vi "RSC_Generate_SubCondition_text.vi"(8 "error in (no error)":errorcluster, 10 "SubCondition #":i32, 11 "Subcondition":refnum<class "Reward_SubCondition.lvclass">) -> (0 "error out":errorcluster, 2 "Validity Criteria":string, 3 "Condition Info":string)   [LabVIEW 2018, in "Tracker.lvlib" / "Reward_SubCondition.lvclass"]
uses:
  Reward_SubCondition.lvclass
  Reward_SubCondition.lvclass/Reward_SubCondition.ctl
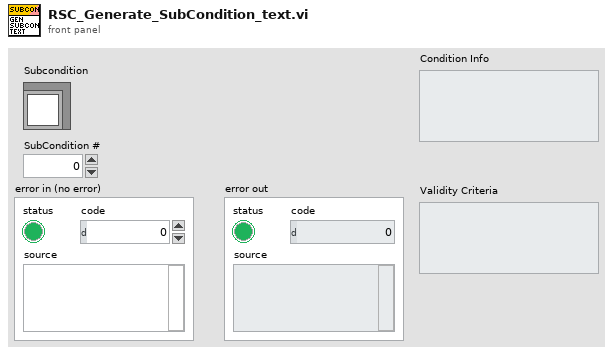
[diagram p1: front panel]
types:
  T1 = enum16{"Less", "Less or Equal", "Equal", "Greater or Equal", "Greater", "Not Equal"}
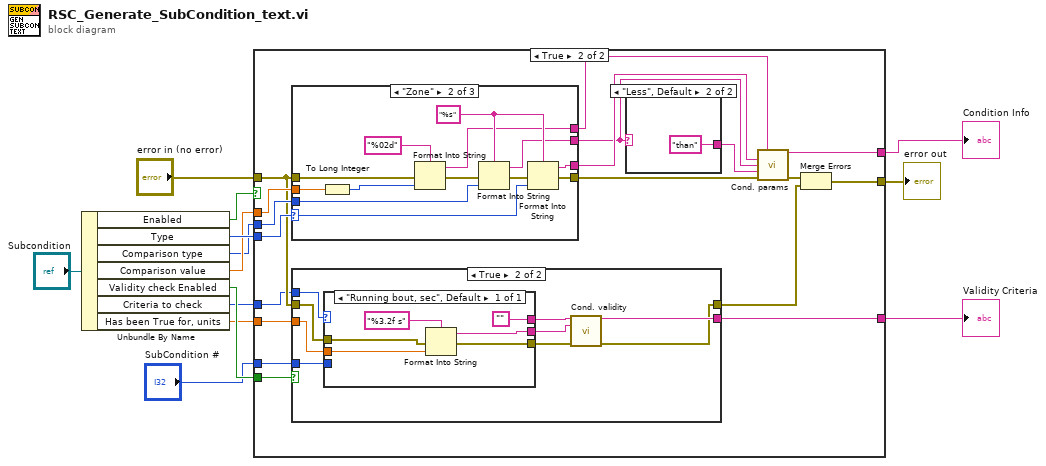
[diagram p0: block diagram]
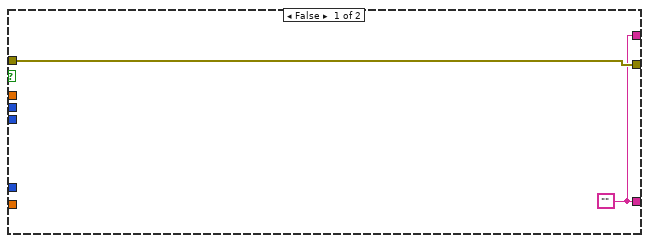
[diagram p2: hidden frame]
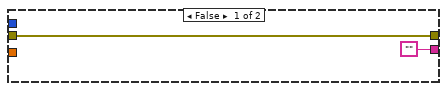
[diagram p3: hidden frame]
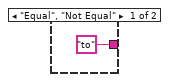
[diagram p4: hidden frame]
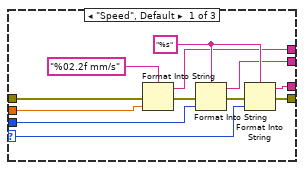
[diagram p5: hidden frame]
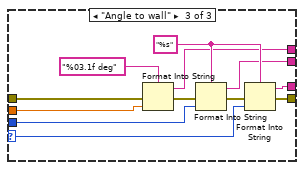
[diagram p6: hidden frame]
diagram:
  n1 = Unbundle By Name("Subcondition") -> ("Enabled"=w7:bool, "Type"=w11:enum16{"Angle to wall", "Speed", "Zone"}, "Comparison type"=w9:T1, "Comparison value"=w10:dbl, "Validity check Enabled"=w8:bool, "Criteria to check"=w4:enum16{"Running bout, sec", "Running bout, m"}, "Has been True for, units"=w5:dbl)
  n2 = case shown="True" w7 {
    tunnel: w11 -> [_ w33]
    tunnel: w10 -> [_ w32]
    tunnel: "error in (no error)" -> [w15 w28]
    tunnel: w9 -> [_ w31]
    tunnel: [w15 w22] -> w12
    tunnel: [w14 w17] -> w1
    tunnel: w8 -> [_ w19]
    tunnel: [w14 w27] -> w2
    tunnel: w5 -> [_ w21]
    tunnel: w4 -> [_ w20]
    tunnel: "SubCondition #" -> [_ w18]
    frame False {
      w14 = ""
    }
    frame True {
      n3 = case shown="\"Zone\"" w33 {
        selector: w33 -> [w62 w75 w88]
        tunnel: w32 -> [w63 w76 w82]
        tunnel: w28 -> [w60 w73 w86]
        tunnel: w31 -> [w61 w74 w87]
        tunnel: [w56 w65 w78] -> w25
        tunnel: [w55 w66 w79] -> w24
        tunnel: [w54 w67 w80] -> w26
        tunnel: [w53 w68 w81] -> w30
        frame "Speed", Default {
          w57 = "%s" ("format string")
          n4 = Format Into String(format string="%02.2f mm/s", error in=w60, w63) -> (resulting string=w54:string, error out=w59:errorcluster)  [unwired: 1 in]
          n5 = Format Into String(format string=w57, error in=w59, w61) -> (resulting string=w55:string, error out=w58:errorcluster)  [unwired: 1 in]
          n6 = Format Into String(format string=w57, error in=w58, w62) -> (resulting string=w56:string, error out=w53:errorcluster)  [unwired: 1 in]
        }
        frame "Zone" {
          w70 = "%s" ("format string")
          n7 = To Long Integer(number=w76) -> (32bit integer=w69:i32)
          n8 = Format Into String(format string="%02d", error in=w73, w69) -> (resulting string=w67:string, error out=w72:errorcluster)  [unwired: 1 in]
          n9 = Format Into String(format string=w70, error in=w72, w74) -> (resulting string=w66:string, error out=w71:errorcluster)  [unwired: 1 in]
          n10 = Format Into String(format string=w70, error in=w71, w75) -> (resulting string=w65:string, error out=w68:errorcluster)  [unwired: 1 in]
        }
        frame "Angle to wall" {
          w83 = "%s" ("format string")
          n11 = Format Into String(format string="%03.1f deg", error in=w86, w82) -> (resulting string=w80:string, error out=w85:errorcluster)  [unwired: 1 in]
          n12 = Format Into String(format string=w83, error in=w85, w87) -> (resulting string=w79:string, error out=w84:errorcluster)  [unwired: 1 in]
          n13 = Format Into String(format string=w83, error in=w84, w88) -> (resulting string=w78:string, error out=w81:errorcluster)  [unwired: 1 in]
        }
      }
      n14 = case shown="True" w19 {
        tunnel: w28 -> [w35 w44]
        tunnel: ["" w43] -> w17
        tunnel: [w35 w42] -> w16
        tunnel: w21 -> [_ w41]
        tunnel: w20 -> [_ w40]
        tunnel: w18 -> [_ w38]
        frame False {
        }
        frame True {
          n15 = case shown="\"Running bout, sec\", Default" w40 {
            tunnel: w44 -> [w48]
            tunnel: w41 -> [w49]
            tunnel: [w45] -> w39
            tunnel: [w47] -> w36
            tunnel: w38 -> [_]
            tunnel: [""] -> w37
            frame "Running bout, sec", Default {
              n16 = Format Into String(format string="%3.2f s", error in=w48, w49) -> (resulting string=w47:string, error out=w45:errorcluster)  [unwired: 1 in]
            }
          }
          n17 = call "Cond. validity"("Beginning Text"=w37, "value"=w36, "error in (no error)"=w39) -> ("Result"=w43:string, "error out"=w42:errorcluster)  [unwired: 11 in]
        }
      }
      n18 = case shown="\"Less\", Default" w24 {
        tunnel: ["to" "than"] -> w23
        frame "Equal", "Not Equal" {
        }
        frame "Less", Default {
        }
      }
      n19 = call "Cond. params"("comvalue"=w26, "condname"=w25, "comptype"=w24, "tie"=w23, "error in (no error)"=w30) -> ("Result"=w27:string, "error out"=w29:errorcluster)  [unwired: 9 in]
      n20 = Merge Errors(w29, w16) -> (w22:errorcluster)
    }
  }
  "error out" <- w12
  "Condition Info" <- w2
  "Validity Criteria" <- w1
